vi "Fetch IQ Recorder Measurement Reliability.vi"(8 "error in (no error)":errorcluster, 10 "Instance (1)":i32=1 format="%.0g", 11 "VISA resource name":refnum<visa-resource-name>) -> (0 "error out":errorcluster, 2 "Reliability Flags":i32[](array[numeric]), 3 "VISA resource name out":refnum<visa-resource-name>)   [LabVIEW 2020, in "Rohde&Schwarz CMXP GPRF.lvlib"]
doc: "Returns the reliability indicator for the I/Q Recorder measurement\n\nAttribute:\nRSCMXPGPRF_ATTR_FETCH_IQ_RECORDER_MEASUREMENT_RELIABILITY\n\nRemote-control command:\nFETCh:GPRF:MEAS<i>:IQRecorder:RELiability?"
uses:
  <instrlib>/Rohde&Schwarz CMXP GPRF/Rohde&Schwarz CMXP GPRF.lvlib
  <instrlib>/Rohde&Schwarz CMXP GPRF/Private/rsidr_core.llb/rsidr_core.lvlib
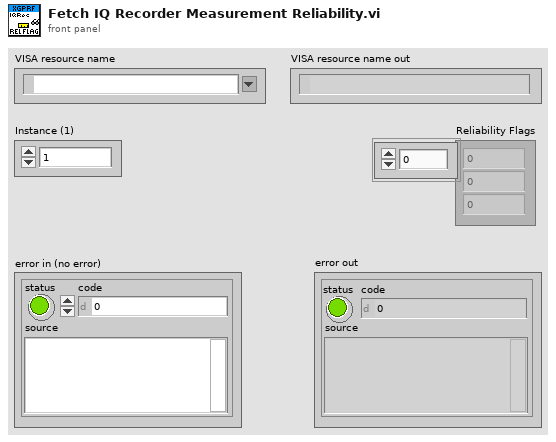
[diagram p1: front panel]
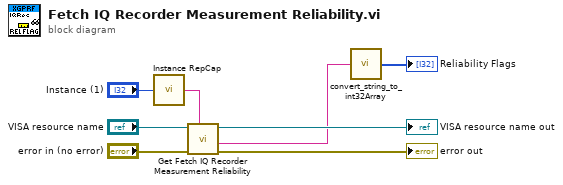
[diagram p0: block diagram]
diagram:
  n1 = call <instrlib>:"Instance RepCap.vi"("Instance in"="Instance (1)") -> ("Instance out"=w3:string)
  n2 = call "Get Fetch IQ Recorder Measurement Reliability"("Repeated Capabilities"=w3, "error in (no error)"="error in (no error)", "instrument handle"="VISA resource name") -> ("error out"=→"error out":errorcluster, "Fetch IQ Recorder Measurement Reliability"=w1:string, "instrument handle out"=→"VISA resource name out":refnum<visa-resource-name>)  [unwired: 6 in]
  n3 = call <instrlib>:"convert_string_to_int32Array.vi"("string in"=w1) -> ("int32 array out"=→"Reliability Flags":i32[])  [unwired: 3 in, 1 out]
